vi "KoherasStatus.vi"() -> ()   [LabVIEW 2011]
panel:
  in  "KoherasStatus":string
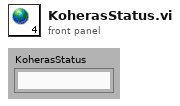
[diagram p1: front panel]
diagram:
